vi "ping.vi"(10 "IP":string) -> (2 "ping结果":bool)   [LabVIEW 2016, in "数据传输系统-05.lvlib" / "自动更新.lvlib" / "TCP文件传输系统.lvlib" / "TCP接收文件.lvlib"]
panel:
  out "匹配子字符串":string
  out "standard output":string caption="标准输出"
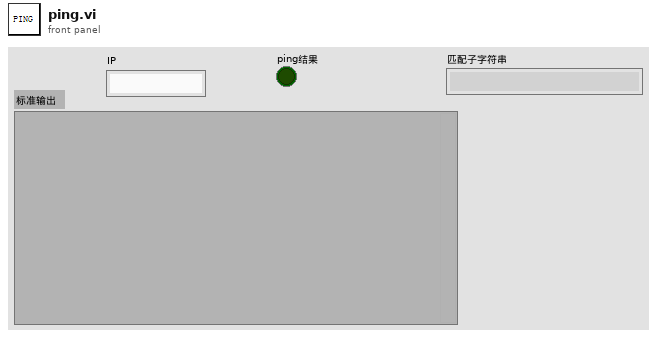
[diagram p1: front panel]
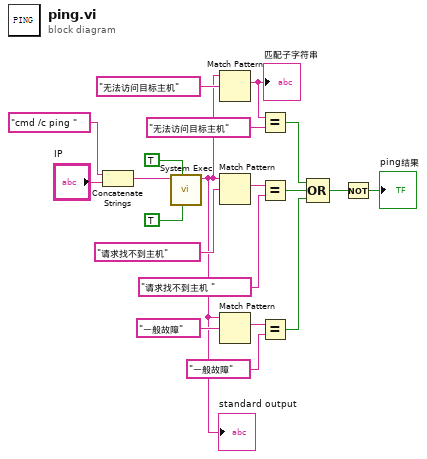
[diagram p0: block diagram]
diagram:
  n1 = Concatenate Strings("cmd /c ping " ("command line"), "IP") -> (w15:string)
  n2 = call <vilib>:"System Exec.vi"("run minimized? (F)"=TRUE, "wait until completion? (T)"=TRUE, "command line"=w15) -> ("standard output"=w2:string)  [unwired: 5 in, 3 out]
  "standard output" <- w2
  n3 = Match Pattern(string=w2, regular expression="无法访问目标主机" ("正则表达式")) -> (match substring=w14:string)  [unwired: 1 in, 3 out]
  "匹配子字符串" <- w14
  n4 = Match Pattern(string=w2, regular expression="请求找不到主机" ("字符串")) -> (match substring=w11:string)  [unwired: 1 in, 3 out]
  n5 = Match Pattern(string=w2, regular expression="一般故障" ("字符串")) -> (match substring=w4:string)  [unwired: 1 in, 3 out]
  n6 = Equal?(x=w14, y="无法访问目标主机" ("正则表达式")) -> (x = y?=w9:bool)
  n7 = Equal?(x=w11, y="请求找不到主机 ") -> (x = y?=w8:bool)
  n8 = Equal?(x=w4, y="一般故障") -> (x = y?=w1:bool)
  n9 = Compound Arithmetic op=OR(w9, w8, w1) -> (w7:bool)
  n10 = Not(x=w7) -> (.not. x?=→"ping结果":bool)
